vi "FGV_HoldingRegs.vi"(6 "FGV_enum":T3=enum."Read", 7 "unit ID":u8=1, 8 "error in (no error)":errorcluster, 9 "FGV_ data cluster":T1, 10 "Instruments":T2=enum."mux10_1(x6)", 11 "Modbus master in":refnum<class "Modbus Master.lvclass">) -> (0 "error out":errorcluster, 2 "HoldingRegs":u16[](array[numeric]), 3 "Modbus master out":refnum<class "Modbus Master.lvclass">)   [LabVIEW 2018, in "MB Relay.lvlib"]
uses:
  MB Relay.lvlib
  type defs/FGV enum.ctl
  <vilib>/NI/Modbus Library/API/Master/Modbus Master.lvclass
  C:/Program Files (x86)/National Instruments/LabVIEW 2018/vi.lib/NI/Modbus Library/API/Modbus API.lvclass
  type defs/MB relays _InstrumentType.ctl
  type defs/FGV data cluster.ctl
  <vilib>/NI/Modbus Library/API/Modbus API.lvclass/Modbus API.ctl
  <vilib>/NI/Modbus Library/Transmission Data Unit/Transmission Data Unit.lvclass/Transmission Data Unit.ctl
  <vilib>/NI/Modbus Library/Transmission Data Unit/Write Unit ID.vi
  <vilib>/NI/Modbus Library/API/Read Transmission Data Unit.vi
  <vilib>/NI/Modbus Library/API/Write Transmission Data Unit.vi
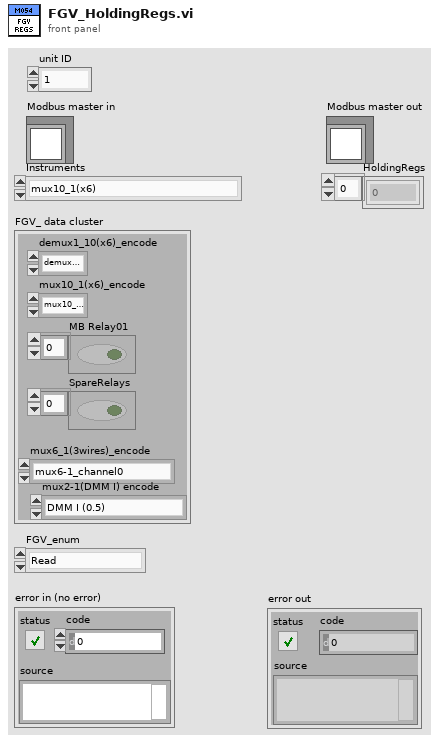
[diagram p1: front panel]
types:
  T1 = typedef "MB Relay.lvlib/FGV data cluster.ctl" = cluster{"demux1_10(x6)_encode":enum16{"demux1_10_channel0", "demux1_10_channel1", "demux1_10_channel2", "demux1_10_channel3", "demux1_10_channel4", "demux1_10_channel5", "demux1_10_channel6", "demux1_10_channel7", "demux1_10_channel8", "demux1_10_channel9", "demux1_10_channel10"}, "mux10_1(x6)_encode":enum16{"mux10_1_channel0", "mux10_1_channel1", "mux10_1_channel2", "mux10_1_channel3", "mux10_1_channel4", "mux10_1_channel5", "mux10_1_channel6", "mux10_1_channel7", "mux10_1_channel8", "mux10_1_channel9", "mux10_1_channel10"}, "MB Relay01":bool[], "SpareRelays":bool[], "mux6_1(3wires)_encode":enum16{"mux6-1_channel0", "mux6_1_channel1_0", "mux6_1_channel1_1", "mux6-1_channel1_2", "mux6_1_channel1_3", "mux6_1_channel2_0", "mux6_1_channel2_1", "mux6_1_channel2_2", "mux6_1_channel2_3", "mux6_1_channel3_0", "mux6_1_channel3_1", "mux6_1_channel3_2", "mux6_1_channel3_3", "mux6_1_channel4_0", "mux6_1_channel4_1", "mux6_1_channel4_2", "mux6_1_channel4_3", "mux6_1_channel5_0", "mux6_1_channel5_1", "mux6_1_channel5_2", "mux6_1_channel5_3", "mux6_1_channel6_0", "mux6_1_channel6_1", "mux6_1_channel6_2", "mux6_1_channel6_3"}, "mux2-1(DMM I) encode":enum16{"DMM I (0.5)", "DMM I (12)"}}
  T2 = typedef "MB Relay.lvlib/MB relays _InstrumentType.ctl" = enum16{"demux1_10(x6)", "mux10_1(x6)", "mux6_1(3wires)", "MB_Relay_01", "SpareRelays", "Optos", "Inputs", "DMM I 0.5"}
  T3 = typedef "MB Relay.lvlib/FGV enum.ctl" = enum16{"Write", "Read", "All OFF", "All ON"}
  T4 = enum16{"demux1_10_channel0", "demux1_10_channel1", "demux1_10_channel2", "demux1_10_channel3", "demux1_10_channel4", "demux1_10_channel5", "demux1_10_channel6", "demux1_10_channel7", "demux1_10_channel8", "demux1_10_channel9", "demux1_10_channel10"}
  T5 = enum16{"mux10_1_channel0", "mux10_1_channel1", "mux10_1_channel2", "mux10_1_channel3", "mux10_1_channel4", "mux10_1_channel5", "mux10_1_channel6", "mux10_1_channel7", "mux10_1_channel8", "mux10_1_channel9", "mux10_1_channel10"}
  T6 = enum16{"mux6-1_channel0", "mux6_1_channel1_0", "mux6_1_channel1_1", "mux6-1_channel1_2", "mux6_1_channel1_3", "mux6_1_channel2_0", "mux6_1_channel2_1", "mux6_1_channel2_2", "mux6_1_channel2_3", "mux6_1_channel3_0", "mux6_1_channel3_1", "mux6_1_channel3_2", "mux6_1_channel3_3", "mux6_1_channel4_0", "mux6_1_channel4_1", "mux6_1_channel4_2", "mux6_1_channel4_3", "mux6_1_channel5_0", "mux6_1_channel5_1", "mux6_1_channel5_2", "mux6_1_channel5_3", "mux6_1_channel6_0", "mux6_1_channel6_1", "mux6_1_channel6_2", "mux6_1_channel6_3"}
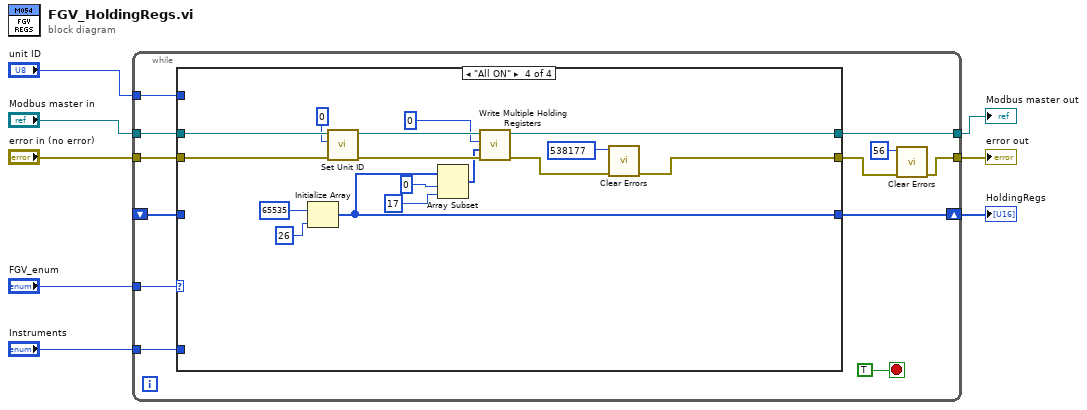
[diagram p0: block diagram]
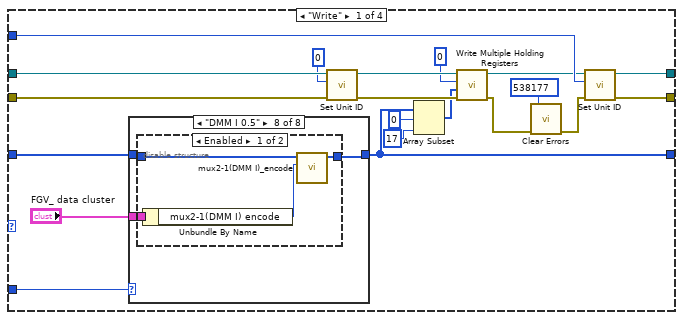
[diagram p2: hidden frame]
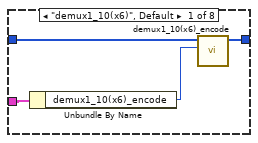
[diagram p3: hidden frame]
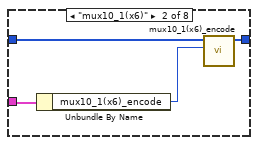
[diagram p4: hidden frame]
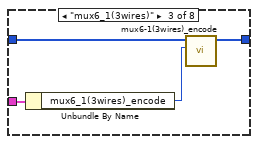
[diagram p5: hidden frame]
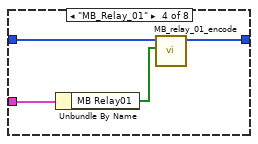
[diagram p6: hidden frame]
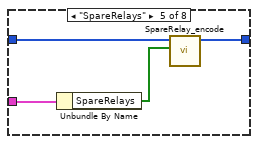
[diagram p7: hidden frame]
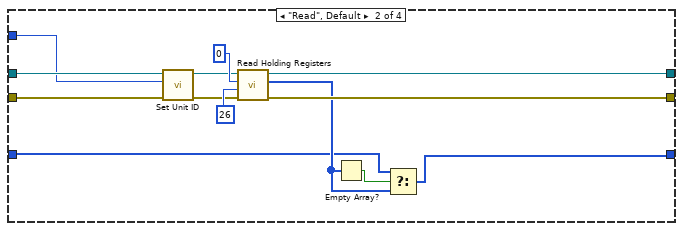
[diagram p11: hidden frame]
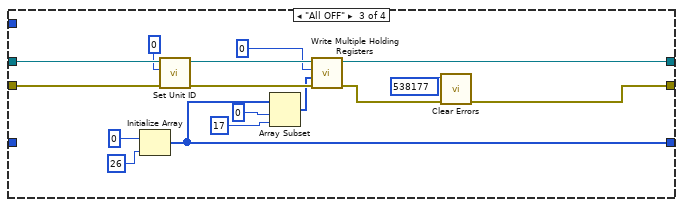
[diagram p12: hidden frame]
diagram:
  n1 = while {
    tunnel: "FGV_enum" -> [w19]
    shift-right: [w18] -> w3
    shift-left: _ -> [w9]
    tunnel: "error in (no error)" -> [w17]
    tunnel: [w12] -> w6
    tunnel: "Modbus master in" -> [w16]
    tunnel: [w15] -> w4
    tunnel: "unit ID" -> [w14]
    tunnel: "Instruments" -> [w10]
    stop <- TRUE stop-if-true
    n2 = case shown="\"All ON\"" w19 {
      tunnel: [w24 w73 w89 w105] -> w18
      tunnel: w17 -> [w40 w80 w97 w113]
      tunnel: [w30 w83 w90 w106] -> w13
      tunnel: w16 -> [w37 w77 w95 w111]
      tunnel: [w32 w76 w93 w109] -> w15
      tunnel: w14 -> [w29 w75 _ _]
      tunnel: w10 -> [w25 _ _ _]
      tunnel: w9 -> [w22 w71 _ _]
      frame "Write" {
        n3 = case shown="\"DMM I 0.5\"" w25 {
          tunnel: w22 -> [w44 w48 w50 w56 w60 w61 w62 w65]
          tunnel: [w43 w47 w51 w55 w59 w61 w62 w64] -> w24
          tunnel: "FGV_ data cluster" -> [w42 w46 w52 w54 w58 _ _ w63]
          frame "demux1_10(x6)", Default {
            n4 = Unbundle By Name(w42) -> ("demux1_10(x6)_encode"=w41:T4)
            n5 = call "demux1_10(x6)_encode.vi"("demux1_10(x6)_encode"=w41, "Mem_mapping in"=w44) -> ("MemMapping Out"=w43:u16[])  [unwired: 8 in, 1 out]
          }
          frame "mux10_1(x6)" {
            n6 = Unbundle By Name(w46) -> ("mux10_1(x6)_encode"=w45:T5)
            n7 = call "mux10_1(x6)_encode.vi"("mux10_1(x6)_encode"=w45, "Mem_mapping in"=w48) -> ("MemMapping Out"=w47:u16[])  [unwired: 8 in, 1 out]
          }
          frame "mux6_1(3wires)" {
            n8 = Unbundle By Name(w52) -> ("mux6_1(3wires)_encode"=w49:T6)
            n9 = call "mux6-1(3wires)_encode.vi"("mux6_1(3wires)_encode"=w49, "Mem_mapping in"=w50) -> ("MemMapping Out"=w51:u16[])  [unwired: 8 in, 1 out]
          }
          frame "MB_Relay_01" {
            n10 = Unbundle By Name(w54) -> ("MB Relay01"=w53:bool[])
            n11 = call "MB_relay_01_encode.vi"("Array"=w53, "Mem_mapping in"=w56) -> ("MemMapping Out"=w55:u16[])  [unwired: 8 in, 1 out]
          }
          frame "SpareRelays" {
            n12 = Unbundle By Name(w58) -> ("SpareRelays"=w57:bool[])
            n13 = call "SpareRelay_encode.vi"("Array"=w57, "Mem_mapping in"=w60) -> ("MemMapping Out"=w59:u16[])  [unwired: 8 in, 1 out]
          }
          frame "Optos" {
          }
          frame "Inputs" {
          }
          frame "DMM I 0.5" {
            n14 = disable-structure shown="Enabled" {
              disable-tunnel: w65 -> [w69 w70]
              disable-tunnel: [w68 w70] -> w64
              disable-tunnel: w63 -> [w67 _]
              frame Enabled {
                n15 = Unbundle By Name(w67) -> ("mux2-1(DMM I) encode"=w66:enum16{"DMM I (0.5)", "DMM I (12)"})
                n16 = call "mux2-1(DMM I)_encode.vi"("mux2-1(DMM I)"=w66, "Mem_mapping in"=w69) -> ("MemMapping Out"=w68:u16[])  [unwired: 8 in, 1 out]
              }
              frame Disabled {
              }
            }
          }
        }
        n17 = call <vilib>:"Set Unit ID.vi"("error in"=w40, "unit ID"=u8 0, "Modbus master in"=w37) -> ("error out"=w39:errorcluster, "Modbus master out"=w38:refnum<class "Modbus Master.lvclass">)  [unwired: 7 in]
        n18 = Array Subset(array=w24, index=0, length=17) -> (w26:u16[])
        n19 = call-dynamic "Write Multiple Holding Registers.vi"("error in"=w39, "registers to write"=w26, "starting address"=u16 0, "Modbus master in"=w38) -> ("error out"=w34:errorcluster, "Modbus master out"=w28:refnum<class "Modbus Master.lvclass">)  [unwired: 6 in]
        n20 = call <vilib>:"Clear Errors.vi"("error in (no error)"=w34, "specific error code to clear (0: all)"=538177) -> ("error out"=w31:errorcluster)  [unwired: 4 in, 1 out]
        n21 = call <vilib>:"Set Unit ID.vi"("error in"=w31, "unit ID"=w29, "Modbus master in"=w28) -> ("error out"=w30:errorcluster, "Modbus master out"=w32:refnum<class "Modbus Master.lvclass">)  [unwired: 7 in]
      }
      frame "Read", Default {
        n22 = call <vilib>:"Set Unit ID.vi"("error in"=w80, "unit ID"=w75, "Modbus master in"=w77) -> ("error out"=w79:errorcluster, "Modbus master out"=w78:refnum<class "Modbus Master.lvclass">)  [unwired: 7 in]
        n23 = call-dynamic "Read Holding Registers.vi"("error in"=w79, "number of inputs"=u16 26, "starting address"=u16 0, "Modbus master in"=w78) -> ("error out"=w83:errorcluster, "register values"=w74:u16[], "Modbus master out"=w76:refnum<class "Modbus Master.lvclass">)  [unwired: 5 in]
        n24 = Empty Array?(array=w74) -> (empty?=w72:bool)
        n25 = Select(t=w71, s=w72, f=w74) -> (s? t:f=w73:u16[])
      }
      frame "All OFF" {
        n26 = Initialize Array(u16 0, 26 ("dimension size")) -> (w89:u16[])
        n27 = call <vilib>:"Set Unit ID.vi"("error in"=w97, "unit ID"=u8 0, "Modbus master in"=w95) -> ("error out"=w96:errorcluster, "Modbus master out"=w94:refnum<class "Modbus Master.lvclass">)  [unwired: 7 in]
        n28 = Array Subset(array=w89, index=0, length=17) -> (w88:u16[])
        n29 = call-dynamic "Write Multiple Holding Registers.vi"("error in"=w96, "registers to write"=w88, "starting address"=u16 0, "Modbus master in"=w94) -> ("error out"=w91:errorcluster, "Modbus master out"=w93:refnum<class "Modbus Master.lvclass">)  [unwired: 6 in]
        n30 = call <vilib>:"Clear Errors.vi"("error in (no error)"=w91, "specific error code to clear (0: all)"=538177) -> ("error out"=w90:errorcluster)  [unwired: 4 in, 1 out]
      }
      frame "All ON" {
        n31 = Initialize Array(u16 65535, 26 ("dimension size")) -> (w105:u16[])
        n32 = call <vilib>:"Set Unit ID.vi"("error in"=w113, "unit ID"=u8 0, "Modbus master in"=w111) -> ("error out"=w112:errorcluster, "Modbus master out"=w110:refnum<class "Modbus Master.lvclass">)  [unwired: 7 in]
        n33 = Array Subset(array=w105, index=0, length=17) -> (w104:u16[])
        n34 = call-dynamic "Write Multiple Holding Registers.vi"("error in"=w112, "registers to write"=w104, "starting address"=u16 0, "Modbus master in"=w110) -> ("error out"=w107:errorcluster, "Modbus master out"=w109:refnum<class "Modbus Master.lvclass">)  [unwired: 6 in]
        n35 = call <vilib>:"Clear Errors.vi"("error in (no error)"=w107, "specific error code to clear (0: all)"=538177) -> ("error out"=w106:errorcluster)  [unwired: 4 in, 1 out]
      }
    }
    n36 = call <vilib>:"Clear Errors.vi"("error in (no error)"=w13, "specific error code to clear (0: all)"=56) -> ("error out"=w12:errorcluster)  [unwired: 4 in, 1 out]
  }
  "error out" <- w6
  "Modbus master out" <- w4
  "HoldingRegs" <- w3
